vi "Get Current.vi"(8 "error in (no error)":errorcluster, 11 "gripper motor_EtherCAT in":refnum<class "NI_Robotics_KUKA youBot Gripper Motor_EtherCAT.lvclass">) -> (0 "error out":errorcluster, 2 "current (A)":dbl, 3 "gripper motor_EtherCAT out":refnum<class "NI_Robotics_KUKA youBot Gripper Motor_EtherCAT.lvclass">)   [LabVIEW 2017, in "NI_Robotics_KUKA youBot Host.lvlib" / "NI_Robotics_KUKA youBot Gripper Motor_EtherCAT.lvclass"]
uses:
  <vilib>/robotics/KUKA youBot/Motor/Gripper Motor EtherCAT/NI_Robotics_KUKA youBot Gripper Motor_EtherCAT.lvclass
  <vilib>/robotics/KUKA youBot/Motor/Gripper Motor EtherCAT/NI_Robotics_KUKA youBot Gripper Motor_EtherCAT.lvclass/NI_Robotics_KUKA youBot Gripper Motor_EtherCAT.ctl
  <vilib>/robotics/KUKA youBot/EtherCAT/EtherCAT Command.ctl
  <vilib>/robotics/KUKA youBot/EtherCAT/CmdCtrls/Param Cmd.ctl
  <vilib>/robotics/KUKA youBot/NI_Robotics_KUKA youBot Host.lvlib
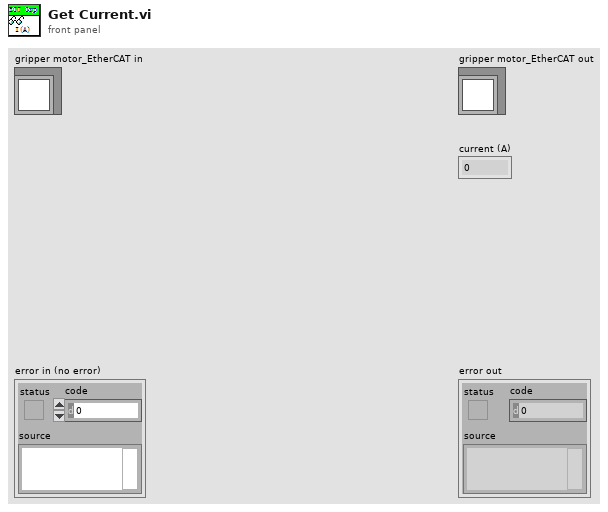
[diagram p1: front panel]
types:
  T1 = typedef "NI_Robotics_KUKA youBot Host.lvlib/EtherCAT Command.ctl" = cluster{"Module":u8, "Cmd":T2, "Type":u8, "Bank":u8, "Val":u32}
  T2 = typedef "NI_Robotics_KUKA youBot Host.lvlib/Param Cmd.ctl" = u8
  T3 = typedef "NI_Robotics_KUKA youBot Host.lvlib/Mater Handler.ctl" = i32
  T4 = typedef "NI_Robotics_KUKA youBot Host.lvlib/EtherCAT Reply.ctl" = cluster{"replyAddr":u8, "moduleAddr":u8, "status":u8, "Cmd":u8, "Val":i32}
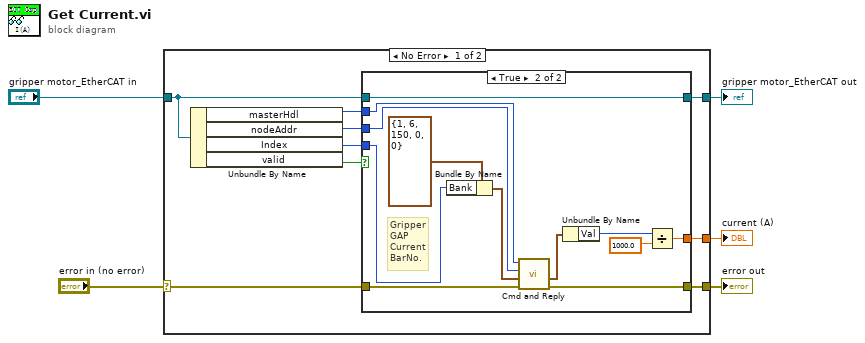
[diagram p0: block diagram]
diagram:
  n1 = case shown="No Error" "error in (no error)" {
    selector: "error in (no error)" -> [w10 w29]
    tunnel: "gripper motor_EtherCAT in" -> [w9 w30]
    tunnel: [w8 _] -> w3
    tunnel: [w7 w30] -> w2
    tunnel: [w6 w29] -> w1
    frame No Error {
      n2 = Unbundle By Name(w9) -> ("masterHdl"=w14:T3, "nodeAddr"=w13:u16, "Index"=w12:i32, "valid"=w11:bool)
      n3 = case shown="True" w11 {
        tunnel: w10 -> [w15 w22]
        tunnel: w9 -> [w16 w21]
        tunnel: w14 -> [_ w28]
        tunnel: w13 -> [_ w27]
        tunnel: w12 -> [_ w25]
        tunnel: [w16 w21] -> w7
        tunnel: [w15 w23] -> w6
        tunnel: [_ w17] -> w8
        frame False {
        }
        frame True {
          # "Gripper\nGAP\nCurrent\nBarNo."
          n4 = Bundle By Name(cluster=T1 {"Module"=1, "Cmd"=6, "Type"=150, "Bank"=0, "Val"=0} ("EtherCAT Command"), "Bank"=w25) -> (w24:T1)
          n5 = call <vilib>:"Cmd and Reply.vi"("error in (no error)"=w22, "EtherCAT command"=w24, "nodeAddr in"=w27, "masterHdl in"=w28) -> ("error out"=w23:errorcluster, "EtherCAT reply"=w20:T4)  [unwired: 3 in, 3 out]
          n6 = Unbundle By Name(w20) -> ("Val"=w19:i32)
          n7 = Divide(x=w19, y=1000.0) -> (x/y=w17:dbl)
        }
      }
    }
    frame Error {
    }
  }
  "error out" <- w1
  "gripper motor_EtherCAT out" <- w2
  "current (A)" <- w3
